vi "sub_Resamp_FSKDemod_Shell.vi"(8 "Rx IQ Sampling\nRate [s/sec]":dbl, 9 "Input Packets":cluster{"Packets":cdb[][], "Enable?":bool}, 10 "FSK Init Parameters":T1) -> (0 "Synch Found?":bool, 1 "Output Bitstream":cluster{"bit stream":i8[][], "Enable?":bool}, 2 "recovered complex waveform":T2[](array[typedef]) {"Y" format="%.3f"; "dt" format="%^.2e"; "t0" format="%.4f"})   [LabVIEW 2015]
uses:
  <vilib>/addons/Modulation/Analog/controls/Complex Data Waveform.ctl
  <vilib>/addons/Modulation/niAMT.lvlib
panel:
  in  "error in (no error)":errorcluster
  out "error out":errorcluster
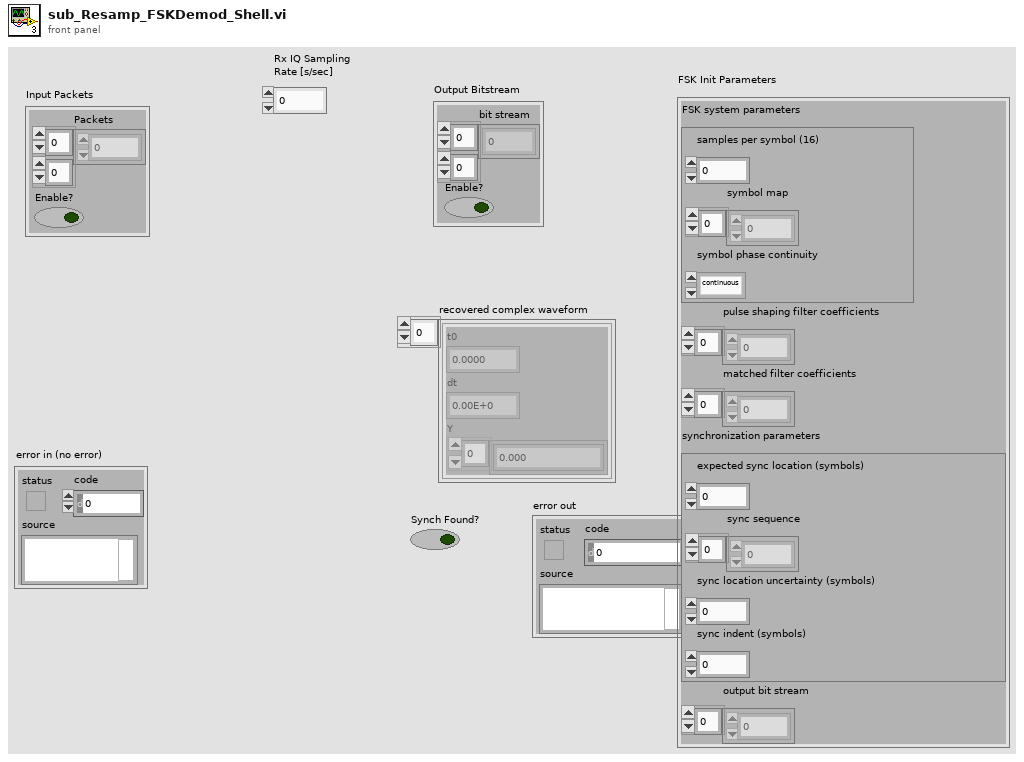
[diagram p1: front panel]
types:
  T1 = cluster{"FSK system parameters":cluster{"samples per symbol (16)":i32, "symbol map":dbl[], "symbol phase continuity":enum16{"continuous", "discontinuous"}}, "pulse shaping filter coefficients":dbl[], "matched filter coefficients":dbl[], "synchronization parameters":cluster{"expected sync location (symbols)":i32, "sync sequence":cdb[], "sync location uncertainty (symbols)":i32, "sync indent (symbols)":i32}, "output bit stream":i8[]}
  T2 = typedef "niAMT.lvlib/Complex Data Waveform.ctl" = cluster{"t0":dbl, "dt":dbl, "Y":cdb[]}
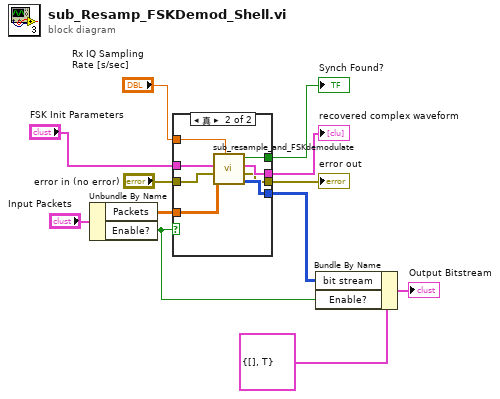
[diagram p0: block diagram]
diagram:
  n1 = Unbundle By Name("Input Packets") -> ("Packets"=w5:cdb[][], "Enable?"=w4:bool)
  n2 = case shown="真" w4 {
    tunnel: "Rx IQ Sampling\nRate [s/sec]" -> [_ w17]
    tunnel: [_ w20] -> w8
    tunnel: [_ w19] -> w7
    tunnel: [_ w18] -> w11
    tunnel: [_ w16] -> w10
    tunnel: "error in (no error)" -> [_ w15]
    tunnel: w5 -> [_ w14]
    tunnel: "FSK Init Parameters" -> [_ w13]
    frame False {
    }
    frame True {
      n3 = call "sub_resample_and_FSKdemodulate.vi"("FSK Init Parameters"=w13, "error in (no error)"=w15, "packet_arr"=w14, "Rx IQ Sampling\nRate [s/sec]"=w17) -> ("Sync Found"=w19:bool, "recovered complex waveform"=w18:T2[], "error out"=w16:errorcluster, "output bit stream"=w20:i8[][])  [unwired: 3 in]
    }
  }
  "Synch Found?" <- w7
  "recovered complex waveform" <- w11
  "error out" <- w10
  n4 = Bundle By Name(cluster=cluster{"bit stream":i8[][], "Enable?":bool} {"bit stream"=[], "Enable?"=TRUE} ("Output Bitstream"), "bit stream"=w8, "Enable?"=w4) -> (→"Output Bitstream":cluster{"bit stream":i8[][], "Enable?":bool})
